vi "Configure Noise Probability Density.vi"(8 "error in (no error)":errorcluster, 9 "Probability Density (0: Gauss 3.1)":u16(ring) items=["Gauss 3.1", "Gauss 4.8", "Gauss 6.0", "Gauss 7.0", "Arbitrary waveform"], 10 "Channel (1: Channel1)":u16(ring) items=["Channel1", "Channel2"], 11 "VISA resource name":refnum<visa-resource-name>) -> (0 "error out":errorcluster, 3 "VISA resource name out":refnum<visa-resource-name>)   [LabVIEW 2009, in "Agilent 81150.lvlib"]
doc: "Configures the probability density function of the noise waveform."
uses:
  Agilent 81150.lvlib
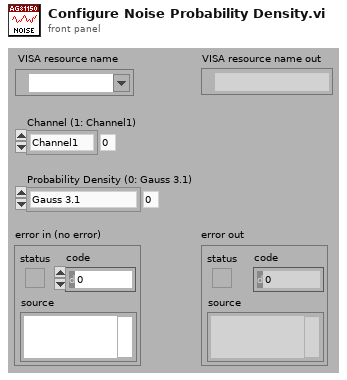
[diagram p1: front panel]
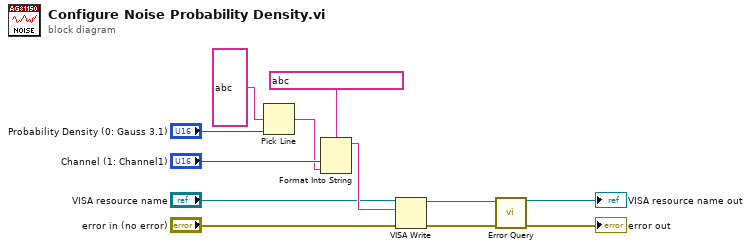
[diagram p0: block diagram]
diagram:
  n1 = Pick Line(multi-line string=string ?, line index="Probability Density (0: Gauss 3.1)") -> (output string=w8:string)  [unwired: 1 out]
  n2 = Format Into String(format string=string ?, "Channel (1: Channel1)", w8) -> (resulting string=w7:string)  [unwired: 2 in, 1 out]
  n3 = VISA Write(VISA resource name="VISA resource name", write buffer=w7, error in (no error)="error in (no error)") -> (VISA resource name out=w4:refnum<visa-resource-name>, error out=w3:errorcluster)  [unwired: 1 out]
  n4 = call "Error Query.vi"("error in (no error)"=w3, "VISA resource name"=w4) -> ("error out"=→"error out":errorcluster, "VISA resource name out"=→"VISA resource name out":refnum<visa-resource-name>)  [unwired: 8 out]
